vi "Set Property.vi"(8 "error in (no error)":errorcluster, 9 "Value":dbl, 10 "Property":string, 11 "Pulse Train in":refnum<class "Pulse Train.lvclass">) -> (0 "error out":errorcluster, 3 "Pulse Train out":refnum<class "Pulse Train.lvclass">)   [LabVIEW 2020, in "Pulse Train.lvclass"]
uses:
  Pulse Train.lvclass
  Pulse Train.lvclass/Pulse Train.ctl
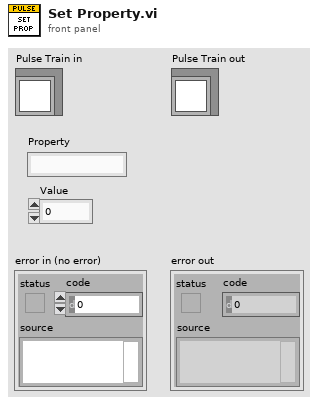
[diagram p1: front panel]
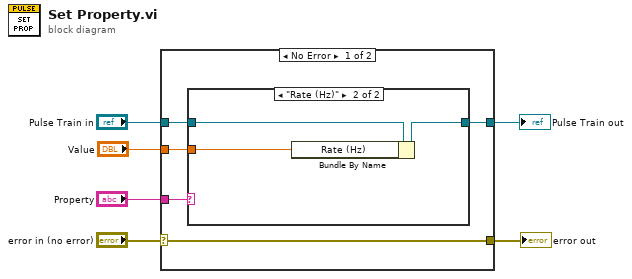
[diagram p0: block diagram]
diagram:
  n1 = case shown="No Error" "error in (no error)" {
    selector: "error in (no error)" -> [w7 w17]
    tunnel: [w7 w17] -> w5
    tunnel: [w9 w16] -> w4
    tunnel: "Pulse Train in" -> [w11 w16]
    tunnel: "Property" -> [w10 _]
    tunnel: "Value" -> [w8 _]
    frame No Error {
      n2 = case shown="\"Rate (Hz)\"" w10 {
        tunnel: w11 -> [w12 w15]
        tunnel: [w12 w14] -> w9
        tunnel: w8 -> [_ w13]
        frame "", Default {
        }
        frame "Rate (Hz)" {
          n3 = Bundle By Name(cluster=w15, "Rate (Hz)"=w13) -> (w14:refnum<class "Pulse Train.lvclass">)
        }
      }
    }
    frame Error {
    }
  }
  "error out" <- w5
  "Pulse Train out" <- w4
